vi "ke37xx Channel Configuration.vi"(0 "VISA Resource Name":refnum<visa-resource-name>, 1 "Channel List":string, 5 "Configuration Name":string, 11 "error in (no error)":errorcluster, 12 "Bytes To Read (1024)":u32=1024) -> (4 "VISA Resource Name Out":refnum<visa-resource-name>, 8 "Configurations":string[](array[string]), 15 "error out":errorcluster)   [LabVIEW 2009, in "Keithley 3700 Series.lvlib"]
doc: "This VI allows you to create or query a measurement configuration associated with a series of channels. You can associate a channel list with the factory default settings for a particular measurement function or with a custom user configuration."
uses:
  <instrlib>/Keithley 3706/Keithley 3700 Series.lvlib
panel:
  in  "Action":enum16{"Set", "Query"}(ring)
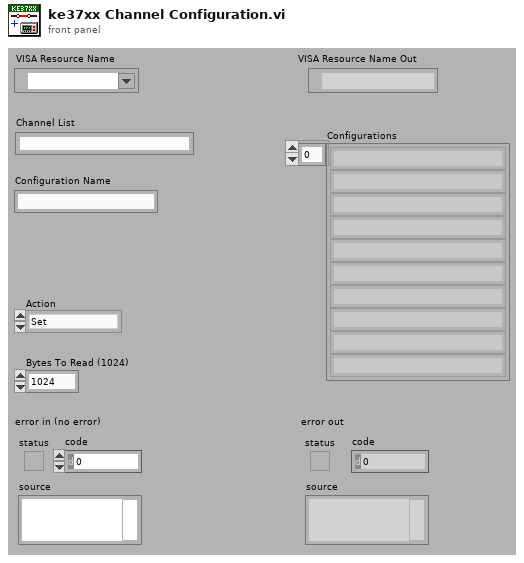
[diagram p1: front panel]
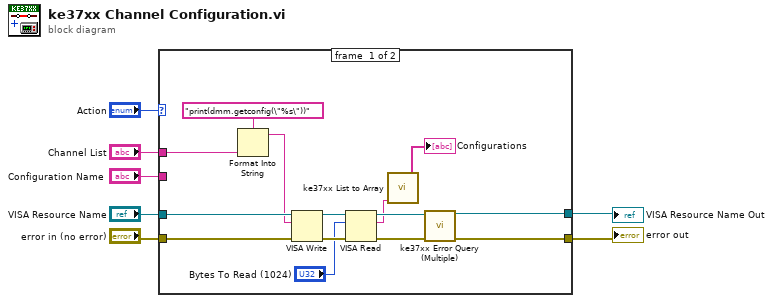
[diagram p0: block diagram]
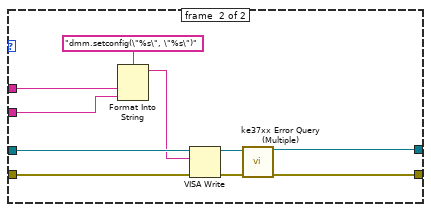
[diagram p2: hidden frame]
diagram:
  n1 = case shown="\"Set\"" "Action" {
    tunnel: [w21 w31] -> w7
    tunnel: [w20 w30] -> w6
    tunnel: "VISA Resource Name" -> [w18 w28]
    tunnel: "error in (no error)" -> [w17 w27]
    tunnel: "Configuration Name" -> [_ w22]
    tunnel: "Channel List" -> [w8 w23]
    frame #0 {
      n2 = Format Into String(format string="print(dmm.getconfig(\"%s\"))", w8) -> (resulting string=w12:string)  [unwired: 2 in, 1 out]
      n3 = VISA Write(VISA resource name=w18, write buffer=w12, error in (no error)=w17) -> (VISA resource name out=w16:refnum<visa-resource-name>, error out=w14:errorcluster)  [unwired: 1 out]
      n4 = VISA Read(VISA resource name=w16, byte count="Bytes To Read (1024)", error in (no error)=w14) -> (VISA resource name out=w15:refnum<visa-resource-name>, read buffer=w10:string, error out=w13:errorcluster)  [unwired: 1 out]
      n5 = call <instrlib>:"ke37xx List to Array.vi"("List"=w10) -> ("Output String Array"=→"Configurations":string[])  [unwired: 1 in, 5 out]
      n6 = call <instrlib>:"ke37xx Error Query (Multiple).vi"("VISA resource name"=w15, "error in (no error)"=w13) -> ("VISA resource name out"=w21:refnum<visa-resource-name>, "error out"=w20:errorcluster)  [unwired: 12 out]
    }
    frame #1 {
      n7 = Format Into String(format string="dmm.setconfig(\"%s\", \"%s\")", w23, w22) -> (resulting string=w26:string)  [unwired: 2 in, 1 out]
      n8 = VISA Write(VISA resource name=w28, write buffer=w26, error in (no error)=w27) -> (VISA resource name out=w25:refnum<visa-resource-name>, error out=w24:errorcluster)  [unwired: 1 out]
      n9 = call <instrlib>:"ke37xx Error Query (Multiple).vi"("VISA resource name"=w25, "error in (no error)"=w24) -> ("VISA resource name out"=w31:refnum<visa-resource-name>, "error out"=w30:errorcluster)  [unwired: 12 out]
    }
  }
  "VISA Resource Name Out" <- w7
  "error out" <- w6
